vi "Day 25 - Full of Hot Air.vi"() -> ()   [LabVIEW 2020, in "AoC 2022.lvlib"]
uses:
  AoC 2022.lvlib
panel:
  in  "Puzzle Input":string="1=-0-2\n12111\n2=0=\n21\n2=01\n111\n20012\n112\n1=-1=\n1-12\n12\n1=\n122"
  out "Puzzle Answer":string
  # "Press Ctrl+M & Enter the Puzzle Input and run the VI"
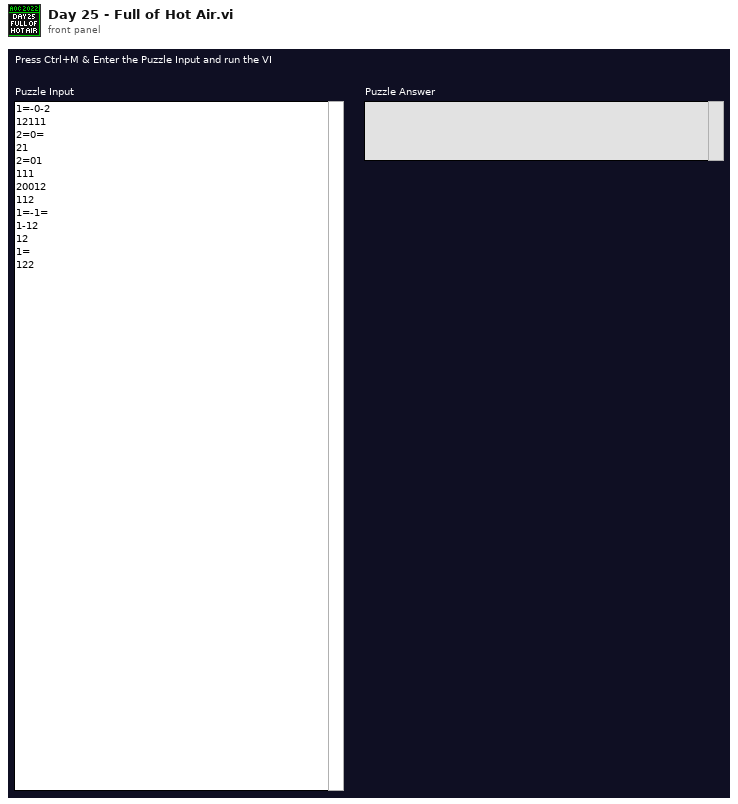
[diagram p1: front panel]
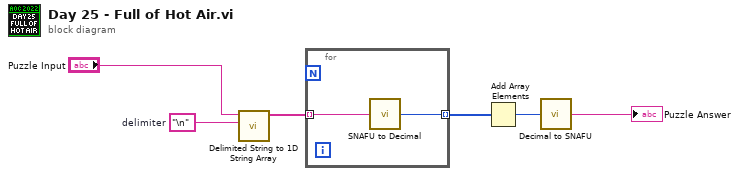
[diagram p0: block diagram]
diagram:
  w5 = "\n"  # delimiter
  n1 = call <vilib>:"Delimited String to 1D String Array.vi"("delimiter"=w5, "delimited string"="Puzzle Input") -> ("string array"=w4:string[])  [unwired: 9 in]
  n2 = for {
    tunnel: w4 -> [w8] mode=indexing
    tunnel: [w7] -> w3 mode=indexing
    n3 = call "SNAFU to Decimal.vi"("SNAFU Number"=w8) -> ("Decimal Number"=w7:i64)
  }
  n4 = Add Array Elements(numeric array=w3) -> (sum=w2:i64)
  n5 = call "Decimal to SNAFU.vi"("Decimal Number"=w2) -> ("SNAFU Number"=→"Puzzle Answer":string)
